vi "GUI_BELLA_ESP-2BL.vi"() -> ()   [LabVIEW 2020]
uses:
  Shared/GUI_Template/GUI_master/tcp_new_data_event.ctl
  Shared/GUI_Template/GUI_master/tcp new data cluster.ctl
panel:
  in  "Position.Axis 4::4":dbl=0.5 caption="M4A Vertical F4" min=-10000.0 max=10000.0 format="%_4f"
  in  "Position.Axis 3::4":dbl=0.5 caption="M4A Horizontal F3" min=-100000.0 max=100000.0 format="%_4f"
  in  "Position.Axis 2::4":dbl=0.5 caption="M2A Vertical F2" min=-10000.0 max=10000.0 format="%_4f"
  in  "Position.Axis 1::4":dbl=0.5 caption="M2A Horizontal F1" min=-100000.0 max=100000.0 format="%_4f"
  in  "Step size 1":dbl=100.0 caption="Step size" min=-22.0 max=22.0
  in  "GUIdevice 4":string="MCD-2BL-M4APicos"
  in  "Status.Axis 3::2":T1(ring) caption="Status"
  in  "Home.Axis 3::2":dbl=0.5 caption="Home" min=0.0 max=6.0 format="%_4f"
  in  "Power.Axis 3::2":enum16{"on", "off"}(ring) caption="Power"
  in  "Position.Axis 3::2":dbl=0.5 caption="Position" min=0.0 max=20.0 format="%_4f"
  in  "Status.Axis 3::3":T1(ring) caption="Status"
  in  "Home.Axis 3::3":dbl=0.5 caption="Home" min=0.0 max=6.0 format="%_4f"
  in  "Power.Axis 3::3":enum16{"on", "off"}(ring) caption="Power"
  in  "Position.Axis 3::3":dbl=0.5 caption="Position" min=0.0 max=20.0 format="%_4f"
  in  "Status.Axis 1::2":T1(ring) caption="Status"
  in  "Home.Axis 1::2":dbl=0.5 caption="Home" min=0.0 max=6.0 format="%_4f"
  in  "Power.Axis 1::2":enum16{"on", "off"}(ring) caption="Power"
  in  "Position.Axis 1::2":dbl=0.5 caption="Position" min=0.0 max=20.0 format="%_4f"
  in  "Status.Axis 2::2":T1(ring) caption="Status"
  in  "Home.Axis 2::2":dbl=0.5 caption="Home" min=0.0 max=6.0 format="%_4f"
  in  "Power.Axis 2::2":enum16{"on", "off"}(ring) caption="Power"
  in  "Position.Axis 2::2":dbl=0.5 caption="Position" min=0.0 max=20.0 format="%_4f"
  in  "Status.Axis 2::3":T1(ring) caption="Status"
  in  "Home.Axis 2::3":dbl=0.5 caption="Home" min=0.0 max=6.0 format="%_4f"
  in  "Power.Axis 2::3":enum16{"on", "off"}(ring) caption="Power"
  in  "Position.Axis 2::3":dbl=0.5 caption="Position" min=0.0 max=20.0 format="%_4f"
  in  "Status.Axis 1::3":T1(ring) caption="Status"
  in  "Home.Axis 1::3":dbl=0.5 caption="Home" min=0.0 max=6.0 format="%_4f"
  in  "Power.Axis 1::3":enum16{"on", "off"}(ring) caption="Power"
  in  "Position.Axis 1::3":dbl=0.5 caption="Position" min=0.0 max=20.0 format="%_4f"
  in  "Status.Axis 1::1":T1(ring) caption="Status"
  in  "Home.Axis 1::1":dbl=0.5 caption="Home" min=0.0 max=6.0 format="%_4f"
  in  "Power.Axis 1::1":enum16{"on", "off"}(ring) caption="Power"
  in  "Position.Axis 1::1":dbl=0.5 caption="Position" min=0.0 max=20.0 format="%_4f"
  in  "Status.Axis 2::1":T1(ring) caption="Status"
  in  "Home.Axis 2::1":dbl=0.5 caption="Home" min=0.0 max=6.0 format="%_4f"
  in  "Power.Axis 2::1":enum16{"on", "off"}(ring) caption="Power"
  in  "Position.Axis 2::1":dbl=0.5 caption="Position" min=0.0 max=20.0 format="%_4f"
  in  "stop":bool
  out "error IO 2":errorcluster
  out "tcp data event":T2
  in  "GUIdevice 3":string="MCD-2BL-ESPBTL3"
  in  "GUIdevice 1":string="MCD-2BL-ESPBTL1"
  in  "GUIdevice 2":string="MCD-2BL-ESPBTL2"
  in  "insert tag":bool=TRUE
  # "BELLA PW 2BL BTL MCD"
  # "F3M2 AXIS 1"
  # "Horizontal"
  # "Vertical"
  # "2BL PICOS"
  # "Horizontal"
  # "Vertical"
  # "F3M6 AXIS 1"
  # "F3M6 AXIS 2"
  # "Horizontal"
  # "Vertical"
  # "F3M5 AXIS 1"
  # "F3M5 AXIS 2"
  # "Horizontal"
  # "Vertical"
  # "F3M3 AXIS 2"
  # "F3M3 AXIS 1"
  # "F3M2 AXIS 2"
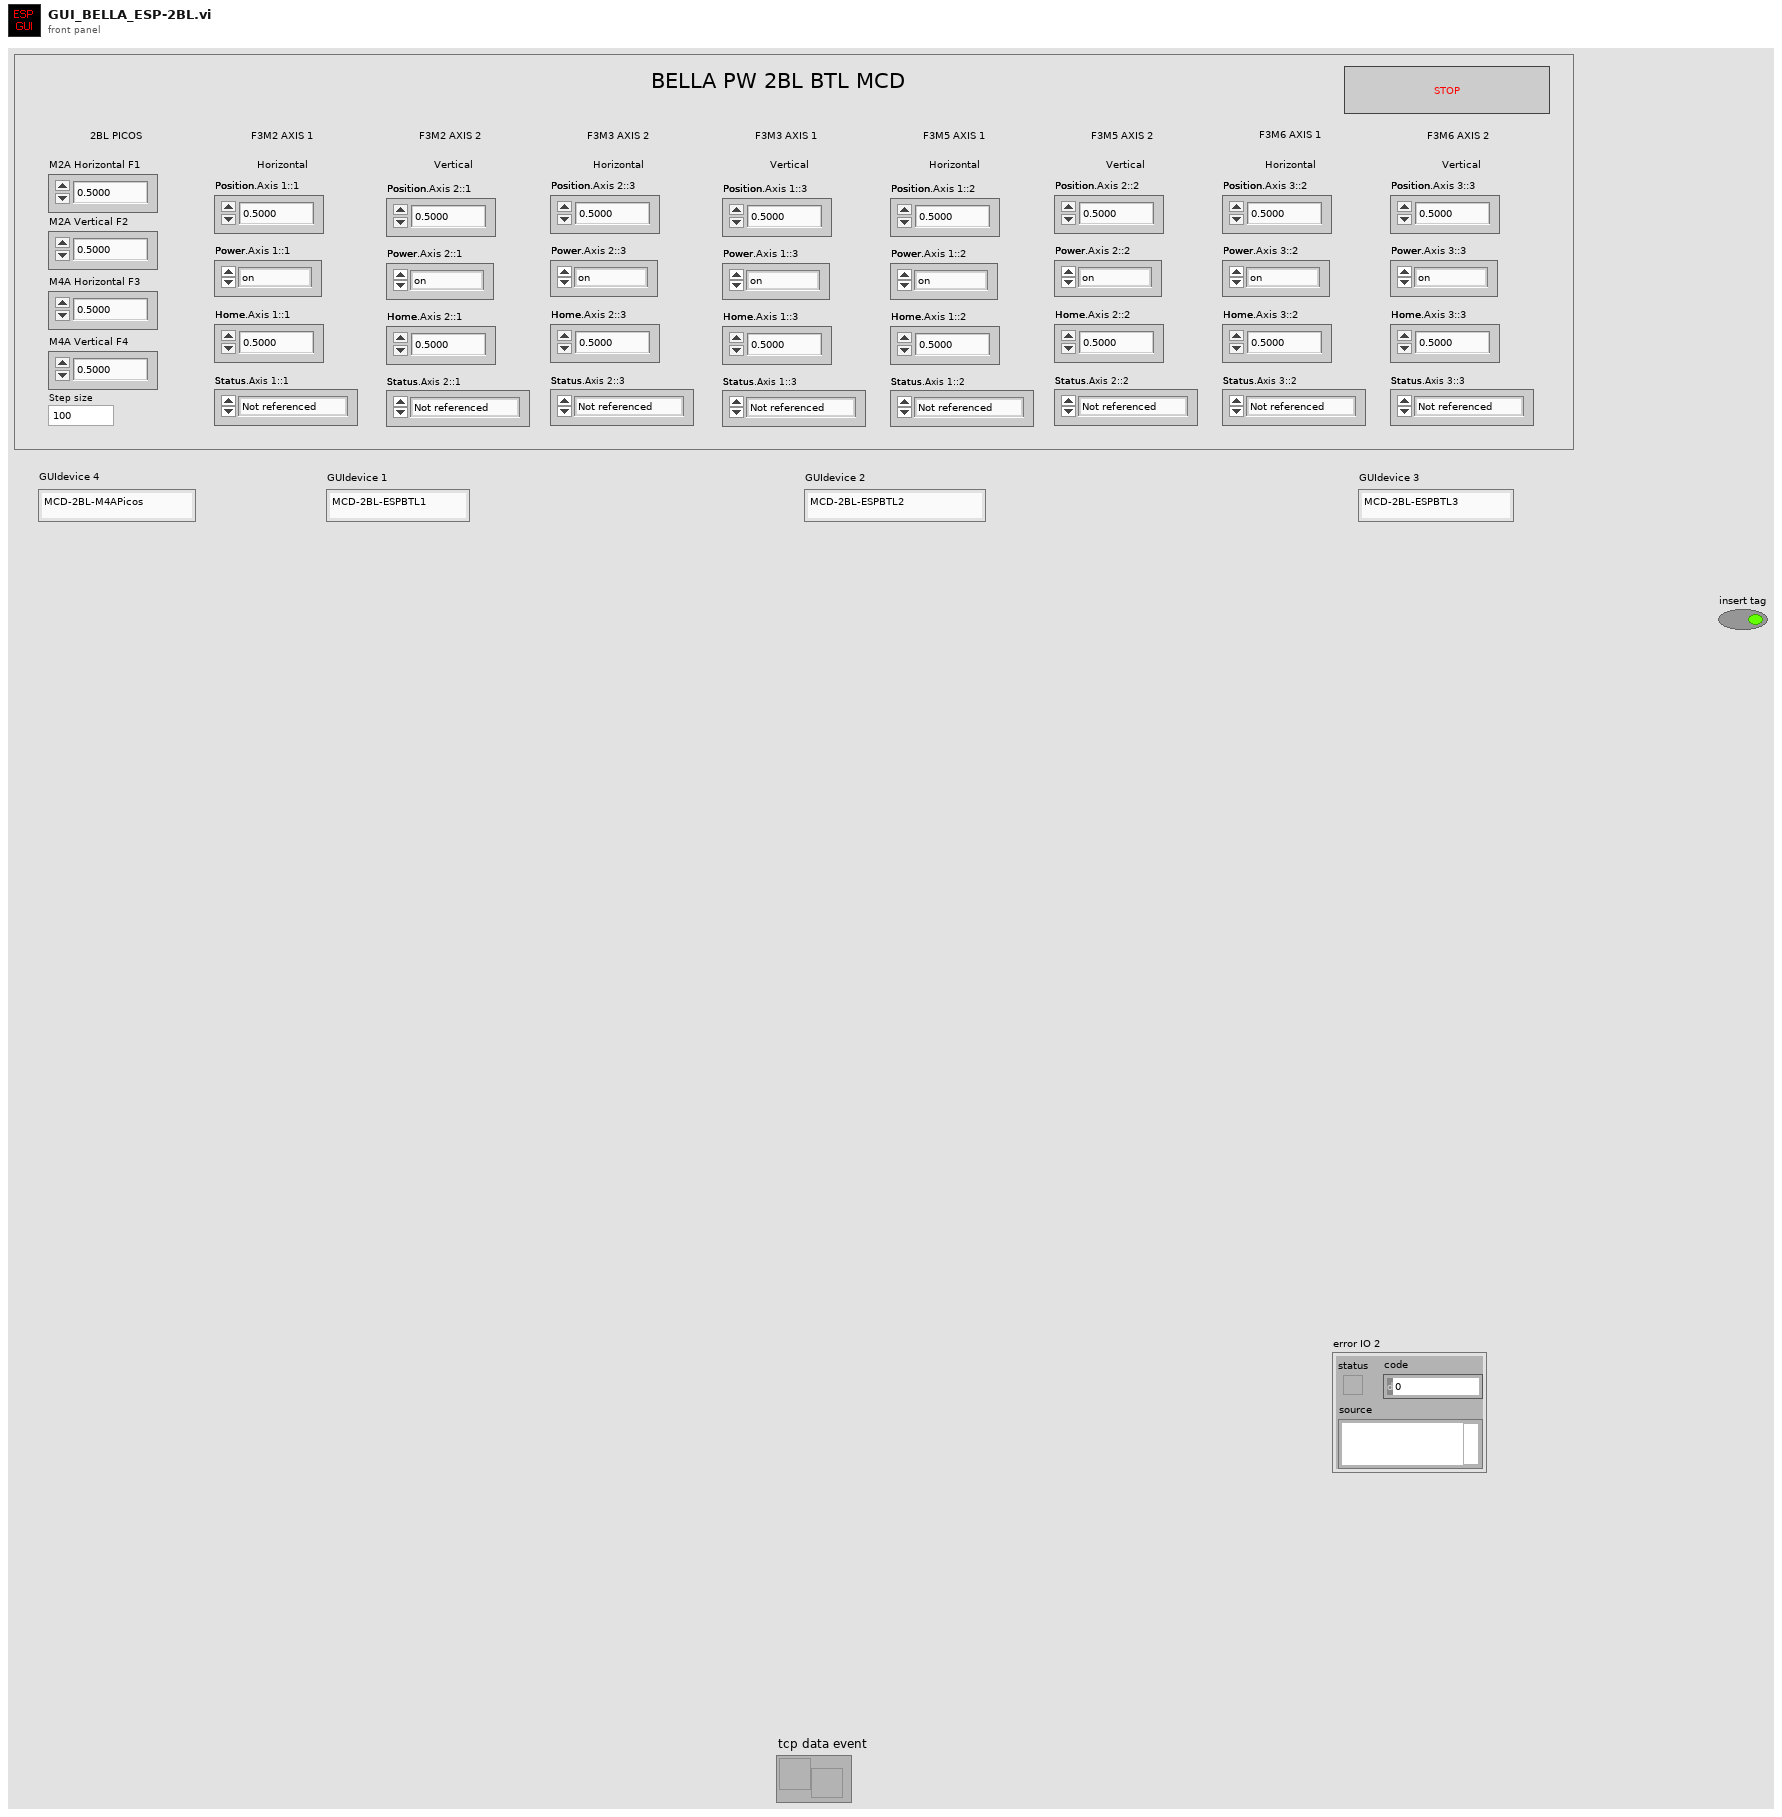
[diagram p1: front panel]
types:
  T1 = enum16{"Not referenced", "Homing", "Moving", "Ready"}
  T2 = typedef "tcp_new_data_event.ctl" = refnum<user-event>
  T3 = typedef "tcp new data cluster.ctl" = cluster{"EventEnum":enum16{"new data", "connection status update"}, "Device name":string}
  T4 = enum32{"Invalid", "Standard", "Closed", "Hidden", "Minimized", "Maximized"}
  T5 = enum32{"invalid app kind", "Development System", "Run Time System", "Student Edition", "Embedded LabVIEW", "Evaluation", "Custom"}
  T6 = cluster{"Core":cluster{"Current VI Reference":refnum<vi>, "Close Panel on Exit?":bool}, "Your Boolean data":bool, "Your string data":string}
  T7 = cluster{"Current VI Reference":refnum<vi>, "Close Panel on Exit?":bool}
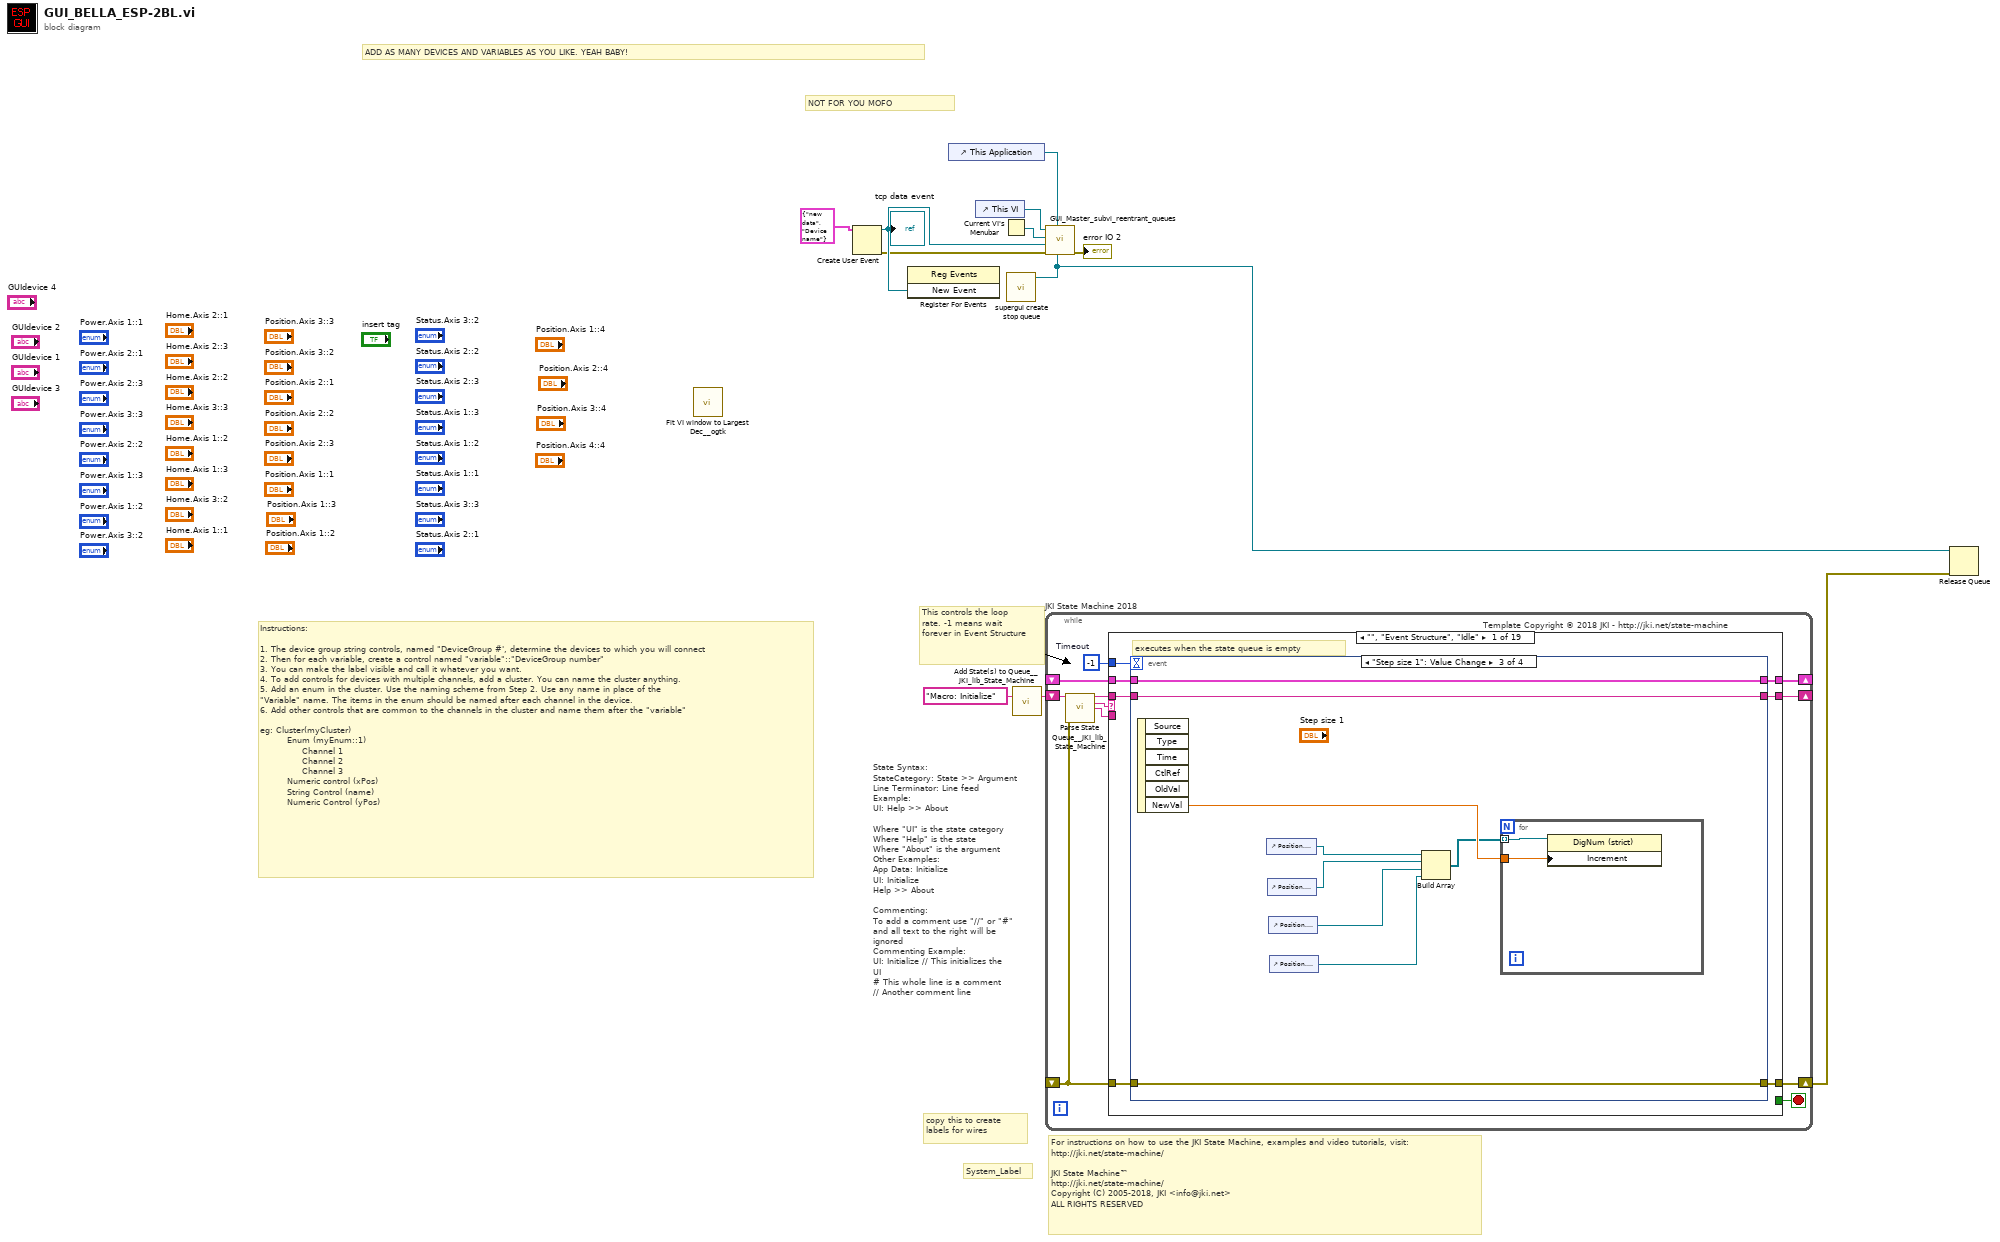
[diagram p0: block diagram]
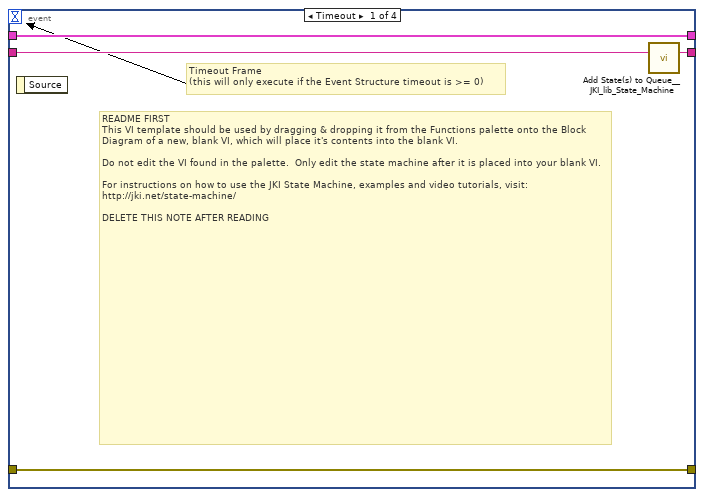
[diagram p2: hidden frame]
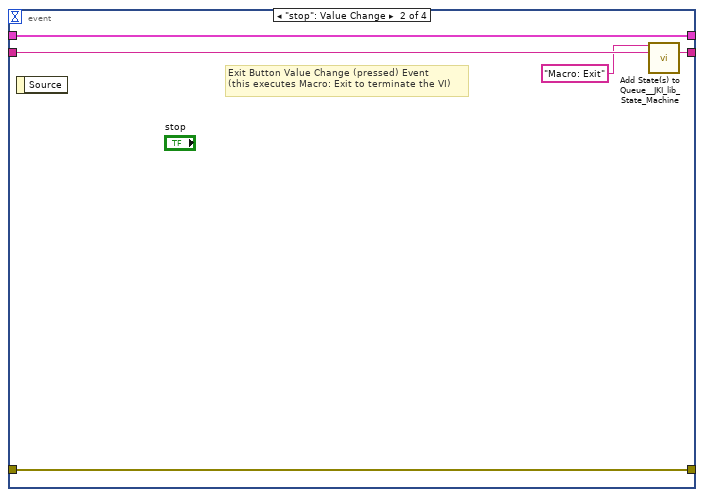
[diagram p3: hidden frame]
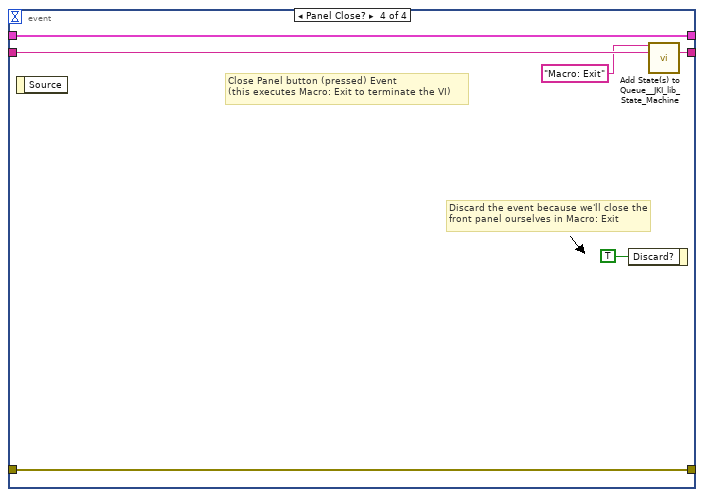
[diagram p4: hidden frame]
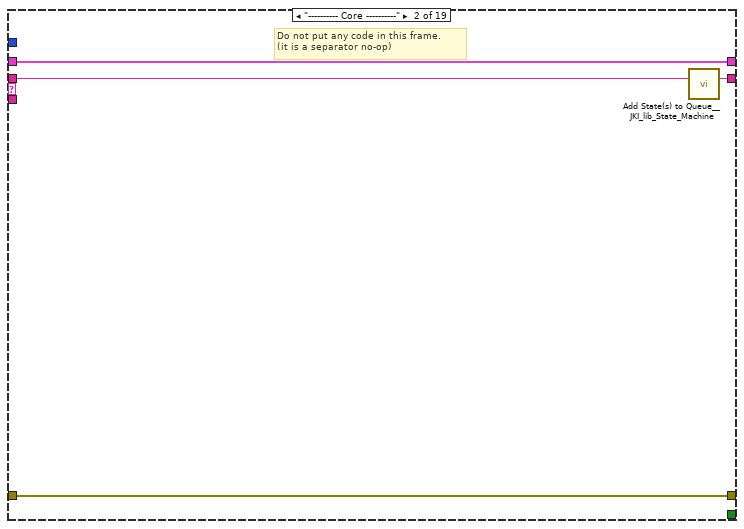
[diagram p5: hidden frame]
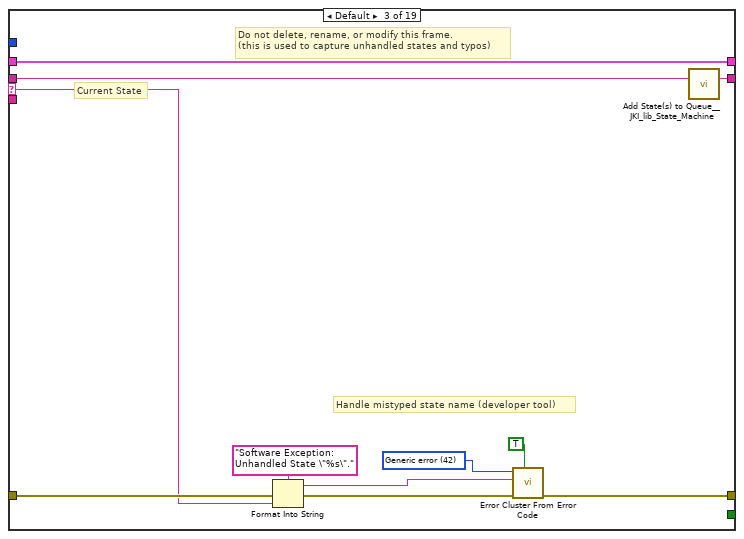
[diagram p6: hidden frame]
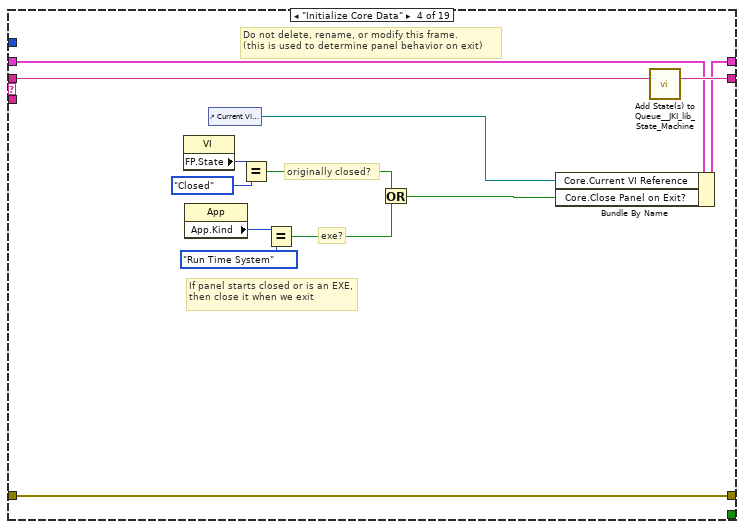
[diagram p7: hidden frame]
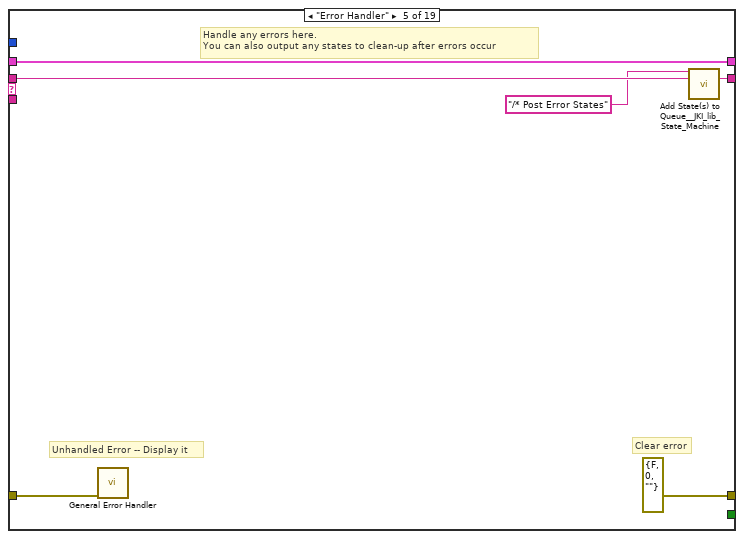
[diagram p8: hidden frame]
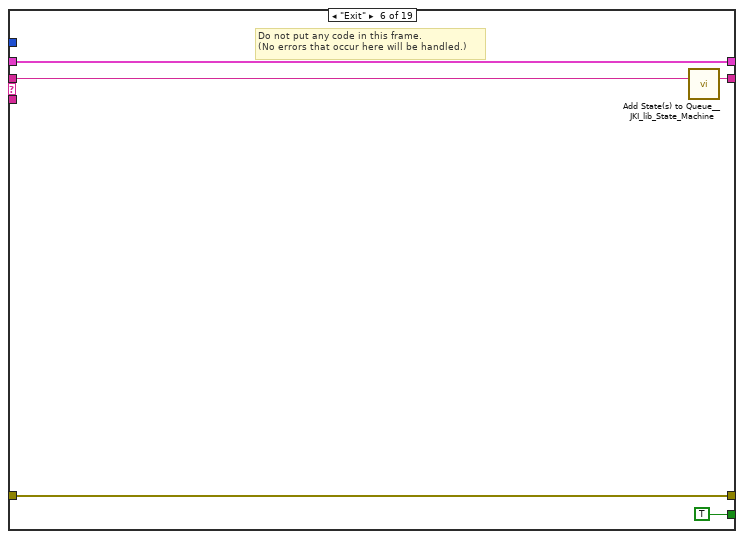
[diagram p9: hidden frame]
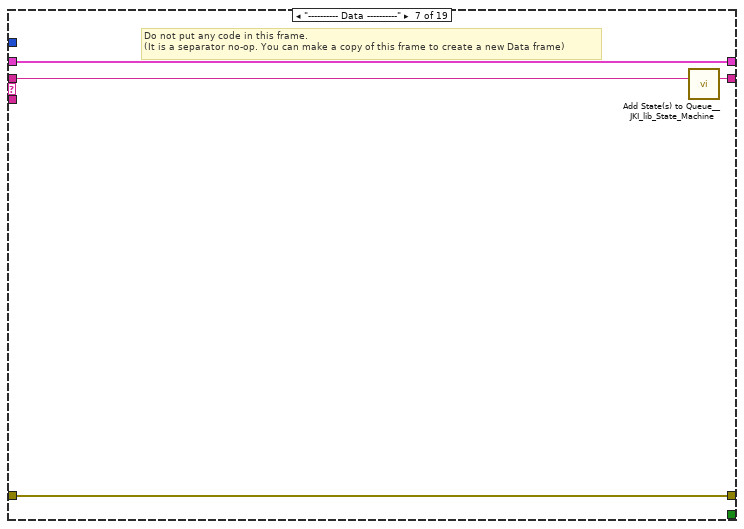
[diagram p10: hidden frame]
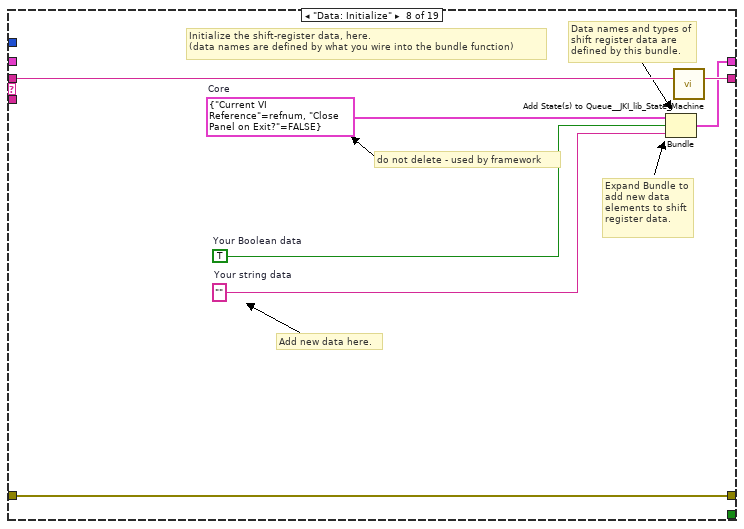
[diagram p11: hidden frame]
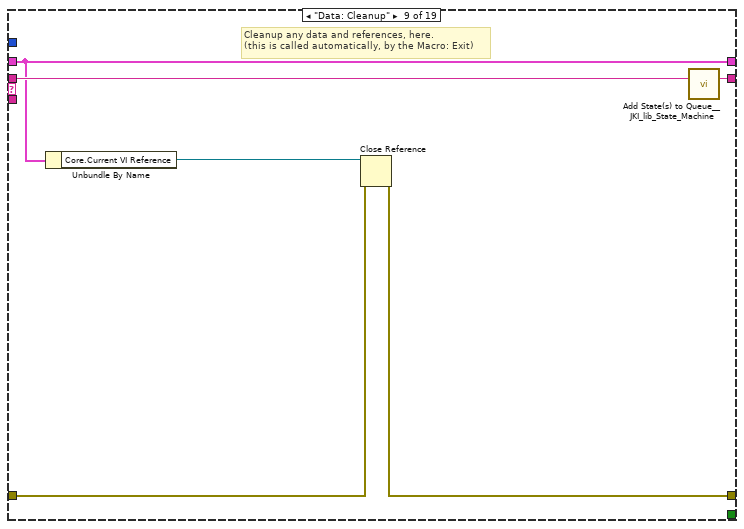
[diagram p12: hidden frame]
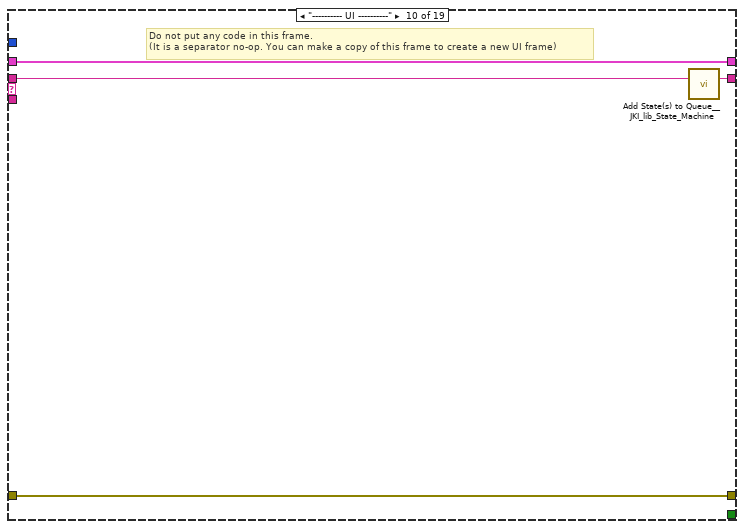
[diagram p13: hidden frame]
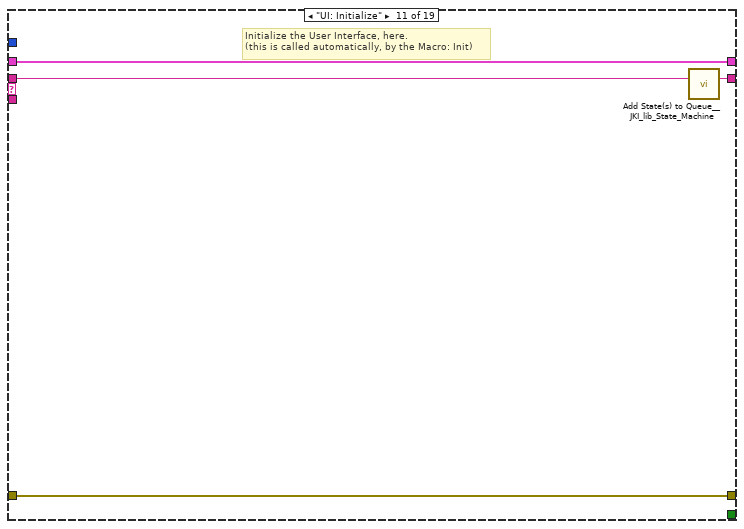
[diagram p14: hidden frame]
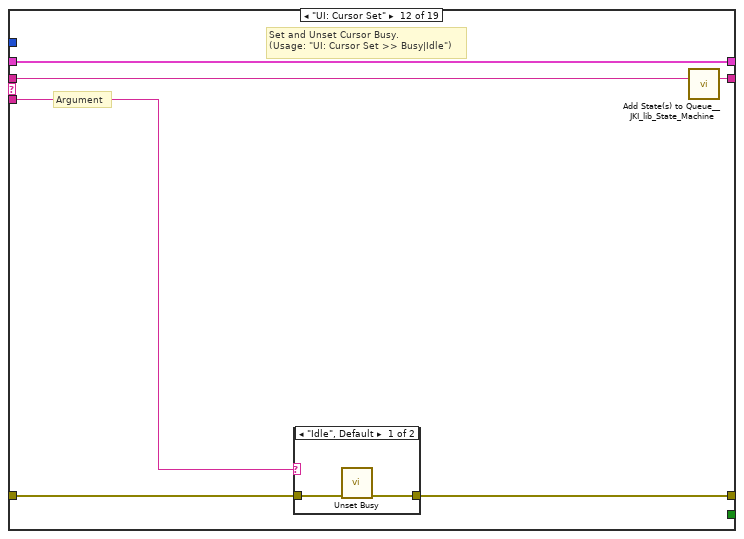
[diagram p15: hidden frame]
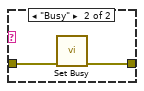
[diagram p16: hidden frame]
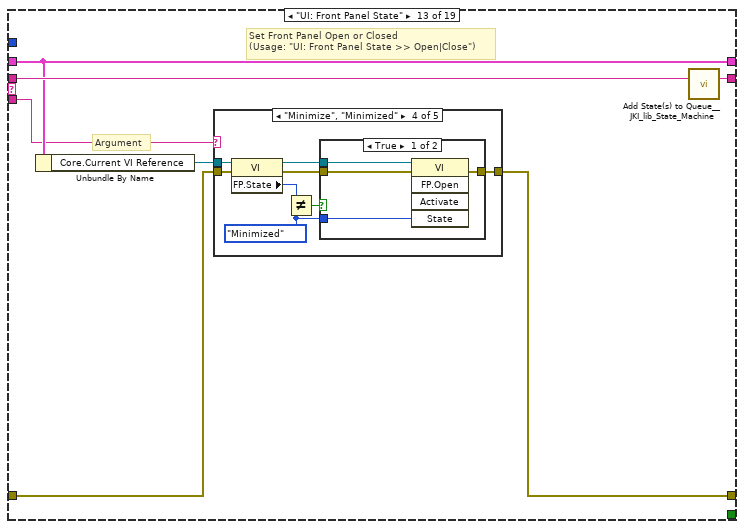
[diagram p17: hidden frame]
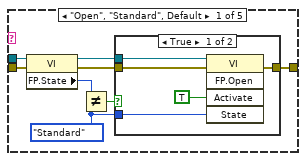
[diagram p18: hidden frame]
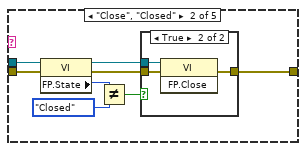
[diagram p20: hidden frame]
diagram:
  # "For instructions on how to use the JKI State Machine, examples and video tutorials, visit:\nhttp://jki.net/state-machine/\n\nJKI State Machine™\nhttp://jki.net/state-machine/\nCopyright (C) 2005-2018, JKI <info@jki.net>\nALL RIGHTS RESERVED"
  # "State Syntax:\nStateCategory: State >> Argument\nLine Terminator: Line feed\nExample:\nUI: Help >> About\n\nWhere \"UI\" is the state category\nWhere \"Help\" is the state\nWhere \"About\" is the argument\nOther Examples:\nApp Data: Initialize\nUI: Initialize\nHelp >> About\n\nCommenting:\nTo add a comment use \"//\" or \"#\" and all text to the right will be ignored\nCommenting Example:\nUI: Initialize // This initializes the UI\n# This whole line is a comment\n// Another comment line"
  # "copy this to create labels for wires"
  # "This controls the loop rate. -1 means wait forever in Event Structure"
  # "System_Label"
  # "NOT FOR YOU MOFO"
  # "Instructions:\n\n1. The device group string controls, named \"DeviceGroup #', determine the devices to which you will connect\n2. Then for each variable, create a control named \"variable\"::\"DeviceGroup number\"\n3. You can make the label visible and call it whatever you want.\n4. To add controls for devices with multiple channels, add a cluster. You can name the cluster anything.\n5. Add an enum in the cluster. Use the naming scheme from Step 2. Use any name in place of the \n\"Variable\" name. The items in the enum should be named after each channel in the device. \n6. Add other controls that are common to the channels in the cluster and name them after the \"variable\"\n\neg: Cluster(myCluster)\n         Enum (myEnum::1)\n              Channel 1 \n              Channel 2\n              Channel 3\n         Numeric control (xPos)\n         String Control (name)\n         Numeric Control (yPos)"
  # "ADD AS MANY DEVICES AND VARIABLES AS YOU LIKE. YEAH BABY!"
  n1 = call <userlib>:"Fit VI window to Largest Dec__ogtk.vi"() -> ()  [unwired: 6 in, 2 out]
  n2 = Create User Event(user event datatype=T3 {"EventEnum"=enum."new data", "Device name"="Device name"} ("New Event")) -> (user event=w10:refnum<user-event>, error out=w9:errorcluster)  [unwired: 1 in]
  "tcp data event" <- w10
  n3 = register-events(w10) -> ()  [unwired: 2 in, 2 out]
  n4 = control-ref of="This Application"() -> (w11:refnum<vi>)
  n5 = control-ref of="This VI"() -> (w6:refnum<vi>)
  n6 = Current VI's Menubar() -> (w7:refnum<k9>)
  n7 = call "supergui create stop queue.vi"() -> ("STOP Queue out"=w4:refnum<queue>)  [unwired: 11 in]
  n8 = call <vilib>:"Add State(s) to Queue__JKI_lib_State_Machine.vi"("State(s) in (\"\")"="Macro: Initialize") -> ("States Out"=w3:string)  [unwired: 14 in]
  n9 = call "GUI_Master_subvi_reentrant_queues.vi"("STOP Queue in"=w4, "This Application"=w11, "error in (no error)"=w9, "tcp data event"=w10, "Caller menu reference"=w7, "Caller VI ref"=w6) -> ("error out"=→"error IO 2":errorcluster)  [unwired: 5 in]
  n10 = while "JKI State Machine 2018" {
    shift-right: [w15] -> _
    shift-left: _ -> [w14]
    shift-right: [w18] -> w1
    shift-left: _ -> [w12]
    shift-right: [w17] -> _
    shift-left: w3 -> [w19]
    stop <- w16 stop-if-true
    w13 = -1  # Timeout
    # "Template Copyright © 2018 JKI - http://jki.net/state-machine"
    n11 = call <vilib>:"Parse State Queue__JKI_lib_State_Machine.vi"("State Queue"=w19, "Error In (no error)"=w12) -> ("Remaining States"=w21:string, "Current State"=w22:string, "Arguments"=w20:string)  [unwired: 11 in]
    n12 = case shown="\"\", \"Event Structure\", \"Idle\"" w22 {
      selector: w22 -> [_ _ w60 _ _ _ _ _ _ _ _ _ _ _ _ _ _ _ _]
      tunnel: w21 -> [w29 w59 w64 w83 w89 w94 w98 w105 w111 w115 w119 w125 w136 w205 w210 w220 w224 w228 w232]
      tunnel: w20 -> [_ _ _ _ _ _ _ _ _ _ _ w120 w130 _ _ _ _ _ _]
      tunnel: w14 -> [w27 w56 w62 w76 w86 w92 w95 _ w106 w112 w117 w123 w132 w202 w207 w217 w221 w225 w229]
      tunnel: [w26 w57 w66 w80 errorcluster {"status"=FALSE, "code"=0, "source"=""} ("error out") w91 w96 w102 w107 w113 w116 w121 w133 w203 w208 w218 w222 w226 w230] -> w18
      tunnel: w12 -> [w25 w57 w65 w80 w85 w91 w96 w102 w108 w113 w116 w122 w134 w203 w208 w218 w222 w226 w230]
      tunnel: [w28 w58 w63 w82 w88 w93 w97 w104 w110 w114 w118 w124 w135 w204 w209 w219 w223 w227 w231] -> w17
      tunnel: [_ _ _ _ _ TRUE _ _ _ _ _ _ _ _ _ _ _ _ _] -> w16
      tunnel: [w24 w56 w62 w81 w86 w92 w95 w103 w106 w112 w117 w123 w132 w202 w207 w217 w221 w225 w229] -> w15
      tunnel: w13 -> [w23 _ _ _ _ _ _ _ _ _ _ _ _ _ _ _ _ _ _]
      frame "", "Event Structure", "Idle" {
        # "executes when the state queue is empty"
        n13 = event shown="[2] \"Step size 1\": Value Change" {
          selector: _ -> [_ _ _ _]
          dyn-events: _ -> [_ _ _ _]
          timeout: w23 -> [_ _ _ _]
          tunnel: w29 -> [w33 w38 w40 w55]
          tunnel: [w32 w37 w40 w54] -> w28
          tunnel: w27 -> [w30 w35 w41 w52]
          tunnel: [w31 w36 w39 w53] -> w26
          tunnel: w25 -> [w31 w36 w39 w53]
          tunnel: [w30 w35 w41 w52] -> w24
          event Timeout {
            # "README FIRST\nThis VI template should be used by dragging & dropping it from the Functions palette onto the Block Diagram of a new, blank VI, which will place it's contents into the blank VI.\n\nDo not edit the VI found in the palette.  Only edit the state machine after it is placed into your blank VI.\n\nFor instructions on how to use the JKI State Machine, examples and video tutorials, visit:\nhttp://jki.net/state-machine/\n\nDELETE THIS NOTE AFTER READING"
            # "Timeout Frame\n(this will only execute if the Event Structure timeout is >= 0)"
            n14 = event-data() -> ()  [unwired: 1 in, 1 out]
            n15 = call <vilib>:"Add State(s) to Queue__JKI_lib_State_Machine.vi"("State(s) in (\"\")"=w33) -> ("States Out"=w32:string)  [unwired: 14 in]
          }
          event "stop": Value Change {
            # "Exit Button Value Change (pressed) Event\n(this executes Macro: Exit to terminate the VI)"
            n16 = event-data() -> ()  [unwired: 1 in, 1 out]
            n17 = call <vilib>:"Add State(s) to Queue__JKI_lib_State_Machine.vi"("State(s) in Front (\"\")"="Macro: Exit", "State(s) in (\"\")"=w38) -> ("States Out"=w37:string)  [unwired: 13 in]
          }
          event "Step size 1": Value Change {
            n18 = event-data() -> ("NewVal"=w43:dbl)  [unwired: 1 in, 5 out]
            n19 = control-ref of="Position.Axis 1::4"() -> (w47:refnum<vi>)
            n20 = control-ref of="Position.Axis 2::4"() -> (w46:refnum<vi>)
            n21 = control-ref of="Position.Axis 3::4"() -> (w45:refnum<vi>)
            n22 = control-ref of="Position.Axis 4::4"() -> (w44:refnum<vi>)
            n23 = Build Array(w47, w46, w45, w44) -> (w42:refnum<vi>[])
            n24 = for {
              tunnel: w43 -> [w49]
              tunnel: w42 -> [w48] mode=indexing
              n25 = property on="Property Node" class="DigNum (strict)"(reference=w48, "Increment"=w49) -> ()  [unwired: 1 in, 2 out]
            }
          }
          event Panel Close? {
            # "Discard the event because we'll close the front panel ourselves in Macro: Exit"
            # "Close Panel button (pressed) Event\n(this executes Macro: Exit to terminate the VI)"
            n26 = event-data() -> ()  [unwired: 1 in, 1 out]
            n27 = event-data("Discard?"=TRUE) -> ()  [unwired: 1 in, 1 out]
            n28 = call <vilib>:"Add State(s) to Queue__JKI_lib_State_Machine.vi"("State(s) in Front (\"\")"="Macro: Exit", "State(s) in (\"\")"=w55) -> ("States Out"=w54:string)  [unwired: 13 in]
          }
        }
      }
      frame "---------- Core ----------" {
        # "Do not put any code in this frame.\n(it is a separator no-op)"
        n29 = call <vilib>:"Add State(s) to Queue__JKI_lib_State_Machine.vi"("State(s) in (\"\")"=w59) -> ("States Out"=w58:string)  [unwired: 14 in]
      }
      frame Default {
        w69 = 42 items=["No error", "Argument error", "Memory is full", "Out of zone", "End of file", "File already open", "Generic file I/O error", "File not found", "File permission error", "Disk is full", "Duplicate path", "Too many files open", "System feature not enabled", "Resource file not found", "Cannot add resource", "Resource not found", "Image not found", "Image memory error", "Pen does not exist", "Config type invalid", "Config token not found", "Config parse error", "Config memory error", "Bad external code format", "Bad external code offset", "External code not present", "Null window", "Destroy window error", "Null menu", "Print aborted", "Bad print record", "Print driver error", "Windows error during printing", "Memory error during printing", "Print dialog error", "Generic print error", "Invalid device refnum", "Device not found", "Device parameter error", "Device unit error", "Cannot open device", "Device call aborted", "Generic error", "Cancelled by user", "Object ID too low", "Object ID too high", "Object not in heap", "Unknown heap", "Unknown object (invalid DefProc)", "Unknown object (DefProc not in table)", "Message out of range", "Invalid (null) method", "Unknown message", "Manager call not supported", "Bad address", "Network operation in progress", "Network operation timed out", "Connection is busy", "Network attribute not supported", "Network error", "Address in use", "System out of memory", "Connection aborted", "Connection refused", "Not connected", "Already connected", "Connection closed", "Initialization error (interapplication manager)", "Bad occurrence", "Wait on unbound occurrence handler", "Occurrence queue overflow", "Datalog type conflict", "Unused", "Unrecognized type (interapplication manager)", "Memory corrupt", "Failed to make temporary DLL", "Old CIN version", "Drag socket not found", "Failed to load drop-object", "Failed to register OLE object", "Failed to release OLE object", "Format specifier type mismatch", "Unknown format specifier", "Too few format specifiers", "Too many format specifiers", "Scan failed", "Newer CIN version", "Error converting to variant", "Runtime menu error", "Password tampered", "Variant attribute not found", "Incompatible variant data type", "Event data is not available", "Event Store is not present", "Occurrence is not found", "Event Queue is not created", "Event info is not available", "Refnum passed is NULL", "Error retrieving Class GUID", "Error retrieving CoClass GUID", "Error retrieving TypeLib GUID.", "Bad built application magic bytes.", "Specific driver is different from the specific driver associated with the Logical Name.", "There is no session opened to the class driver.", "Max Error", "MAX - Error with config objects", "MAX - Error loading configuration", "MAX - Group not supported"]
        # "Current State"
        # "Do not delete, rename, or modify this frame.\n(this is used to capture unhandled states and typos)"
        # "Handle mistyped state name (developer tool)"
        n30 = Format Into String(format string="Software Exception: Unhandled State \"%s\"." ("message"), error in=w65, w60) -> (resulting string=w68:string, error out=w67:errorcluster)  [unwired: 1 in]
        n31 = call <vilib>:"Error Cluster From Error Code.vi"("show call chain? (False)"=TRUE, "error in (no error)"=w67, "error message (\"\")"=w68, "error code (0)"=w69) -> ("error out"=w66:errorcluster)  [unwired: 5 in]
        n32 = call <vilib>:"Add State(s) to Queue__JKI_lib_State_Machine.vi"("State(s) in (\"\")"=w64) -> ("States Out"=w63:string)  [unwired: 14 in]
      }
      frame "Initialize Core Data" {
        # "Do not delete, rename, or modify this frame.\n(this is used to determine panel behavior on exit)"
        # "originally closed?"
        # "exe?"
        # "If panel starts closed or is an EXE, then close it when we exit"
        n33 = property class="VI"() -> ("FP.State"=w73:T4)  [unwired: 2 in, 2 out]
        n34 = property class="App"() -> ("App.Kind"=w79:T5)  [unwired: 2 in, 2 out]
        n35 = control-ref of="Current VI Reference"() -> (w74:refnum<vi>)
        n36 = Equal?(x=w73, y=T4."Closed" ("Front Panel Window:State")) -> (x = y?=w71:bool)
        n37 = Equal?(x=w79, y=T5."Run Time System" ("Application:Kind")) -> (x = y?=w77:bool)
        n38 = Or(x=w71, y=w77) -> (x .or. y?=w75:bool)
        n39 = Bundle By Name(cluster=w76, "Core.Current VI Reference"=w74, "Core.Close Panel on Exit?"=w75) -> (w81:T6)
        n40 = call <vilib>:"Add State(s) to Queue__JKI_lib_State_Machine.vi"("State(s) in (\"\")"=w83) -> ("States Out"=w82:string)  [unwired: 14 in]
      }
      frame "Error Handler" {
        # "Unhandled Error -- Display it"
        # "Handle any errors here.\nYou can also output any states to clean-up after errors occur"
        # "Clear error"
        n41 = call <vilib>:"General Error Handler.vi"("error in (no error)"=w85) -> ()  [unwired: 10 in, 5 out]
        n42 = call <vilib>:"Add State(s) to Queue__JKI_lib_State_Machine.vi"("State(s) in Front (\"\")"="/* Post Error States", "State(s) in (\"\")"=w89) -> ("States Out"=w88:string)  [unwired: 13 in]
      }
      frame "Exit" {
        # "Do not put any code in this frame.\n(No errors that occur here will be handled.)"
        n43 = call <vilib>:"Add State(s) to Queue__JKI_lib_State_Machine.vi"("State(s) in (\"\")"=w94) -> ("States Out"=w93:string)  [unwired: 14 in]
      }
      frame "---------- Data ----------" {
        # "Do not put any code in this frame.\n(It is a separator no-op. You can make a copy of this frame to create a new Data frame)"
        n44 = call <vilib>:"Add State(s) to Queue__JKI_lib_State_Machine.vi"("State(s) in (\"\")"=w98) -> ("States Out"=w97:string)  [unwired: 14 in]
      }
      frame "Data: Initialize" {
        w99 = T7 {"Current VI Reference"=refnum, "Close Panel on Exit?"=FALSE}  # Core
        w101 = TRUE  # Your Boolean data
        w100 = ""  # Your string data
        # "do not delete - used by framework"
        # "Expand Bundle to add new data elements to shift register data."
        # "Add new data here."
        # "Data names and types of shift register data are defined by this bundle."
        # "Initialize the shift-register data, here.\n(data names are defined by what you wire into the bundle function)"
        n45 = Bundle("Core"=w99, "Your Boolean data"=w101, "Your string data"=w100) -> (w103:T6)  [unwired: 1 in]
        n46 = call <vilib>:"Add State(s) to Queue__JKI_lib_State_Machine.vi"("State(s) in (\"\")"=w105) -> ("States Out"=w104:string)  [unwired: 14 in]
      }
      frame "Data: Cleanup" {
        # "Cleanup any data and references, here.\n(this is called automatically, by the Macro: Exit)"
        n47 = Unbundle By Name(w106) -> ("Core.Current VI Reference"=w109:refnum<vi>)
        n48 = Close Reference(reference=w109, error in (no error)=w108) -> (error out=w107:errorcluster)
        n49 = call <vilib>:"Add State(s) to Queue__JKI_lib_State_Machine.vi"("State(s) in (\"\")"=w111) -> ("States Out"=w110:string)  [unwired: 14 in]
      }
      frame "---------- UI ----------" {
        # "Do not put any code in this frame.\n(It is a separator no-op. You can make a copy of this frame to create a new UI frame)"
        n50 = call <vilib>:"Add State(s) to Queue__JKI_lib_State_Machine.vi"("State(s) in (\"\")"=w115) -> ("States Out"=w114:string)  [unwired: 14 in]
      }
      frame "UI: Initialize" {
        # "Initialize the User Interface, here.\n(this is called automatically, by the Macro: Init)"
        n51 = call <vilib>:"Add State(s) to Queue__JKI_lib_State_Machine.vi"("State(s) in (\"\")"=w119) -> ("States Out"=w118:string)  [unwired: 14 in]
      }
      frame "UI: Cursor Set" {
        # "Argument"
        # "Set and Unset Cursor Busy.\n(Usage: \"UI: Cursor Set >> Busy|Idle\")"
        n52 = case shown="\"Idle\", Default" w120 {
          tunnel: w122 -> [w127 w129]
          tunnel: [w126 w128] -> w121
          frame "Idle", Default {
            n53 = call <vilib>:"Unset Busy.vi"("error in (no error)"=w127) -> ("error out"=w126:errorcluster)  [unwired: 10 in]
          }
          frame "Busy" {
            n54 = call <vilib>:"Set Busy.vi"("error in (no error)"=w129) -> ("error out"=w128:errorcluster)  [unwired: 9 in, 1 out]
          }
        }
        n55 = call <vilib>:"Add State(s) to Queue__JKI_lib_State_Machine.vi"("State(s) in (\"\")"=w125) -> ("States Out"=w124:string)  [unwired: 14 in]
      }
      frame "UI: Front Panel State" {
        # "Argument"
        # "Set Front Panel Open or Closed\n(Usage: \"UI: Front Panel State >> Open|Close\")"
        n56 = Unbundle By Name(w132) -> ("Core.Current VI Reference"=w131:refnum<vi>)
        n57 = case shown="\"Minimize\", \"Minimized\"" w130 {
          tunnel: w134 -> [w142 w157 w168 w181 w194]
          tunnel: [w144 w158 w170 w183 w196] -> w133
          tunnel: w131 -> [w143 w155 w169 w182 w195]
          frame "Open", "Standard", Default {
            w137 = T4."Standard" ("State")
            n58 = property class="VI"(reference=w143, error in=w142) -> (reference out=w140:refnum<vi>, error out=w141:errorcluster, "FP.State"=w139:T4)
            n59 = Not Equal?(x=w139, y=w137) -> (x != y?=w138:bool)
            n60 = case shown="True" w138 {
              tunnel: [w148 w150] -> w144
              tunnel: w141 -> [w147 w150]
              tunnel: w140 -> [w146 _]
              tunnel: w137 -> [w145 _]
              frame True {
                n61 = invoke class="VI" method="FP.Open"(reference=w146, error in=w147, "Activate"=TRUE, "State"=w145) -> (error out=w148:errorcluster)  [unwired: 1 in, 4 out]
              }
              frame False {
              }
            }
          }
          frame "Close", "Closed" {
            n62 = property class="VI"(reference=w155, error in=w157) -> (reference out=w154:refnum<vi>, error out=w156:errorcluster, "FP.State"=w152:T4)
            n63 = Not Equal?(x=w152, y=T4."Closed" ("Front Panel Window:State")) -> (x != y?=w151:bool)
            n64 = case shown="True" w151 {
              tunnel: [w159 w162] -> w158
              tunnel: w156 -> [w159 w161]
              tunnel: w154 -> [_ w160]
              frame False {
              }
              frame True {
                n65 = invoke class="VI" method="FP.Close"(reference=w160, error in=w161) -> (error out=w162:errorcluster)  [unwired: 1 in, 2 out]
              }
            }
          }
          frame "Hidden", "Hide" {
            w163 = T4."Hidden" ("State")
            n66 = property class="VI"(reference=w169, error in=w168) -> (reference out=w166:refnum<vi>, error out=w167:errorcluster, "FP.State"=w165:T4)
            n67 = Not Equal?(x=w165, y=w163) -> (x != y?=w164:bool)
            n68 = case shown="True" w164 {
              tunnel: [w174 w175] -> w170
              tunnel: w167 -> [w173 w175]
              tunnel: w166 -> [w172 _]
              tunnel: w163 -> [w171 _]
              frame True {
                n69 = invoke class="VI" method="FP.Open"(reference=w172, error in=w173, "State"=w171) -> (error out=w174:errorcluster)  [unwired: 2 in, 4 out]
              }
              frame False {
              }
            }
          }
          frame "Minimize", "Minimized" {
            w176 = T4."Minimized" ("State")
            n70 = property class="VI"(reference=w182, error in=w181) -> (reference out=w179:refnum<vi>, error out=w180:errorcluster, "FP.State"=w178:T4)
            n71 = Not Equal?(x=w178, y=w176) -> (x != y?=w177:bool)
            n72 = case shown="True" w177 {
              tunnel: [w187 w188] -> w183
              tunnel: w180 -> [w186 w188]
              tunnel: w179 -> [w185 _]
              tunnel: w176 -> [w184 _]
              frame True {
                n73 = invoke class="VI" method="FP.Open"(reference=w185, error in=w186, "State"=w184) -> (error out=w187:errorcluster)  [unwired: 2 in, 4 out]
              }
              frame False {
              }
            }
          }
          frame "Maximize", "Maximized" {
            w189 = T4."Maximized" ("State")
            n74 = property class="VI"(reference=w195, error in=w194) -> (reference out=w192:refnum<vi>, error out=w193:errorcluster, "FP.State"=w191:T4)
            n75 = Not Equal?(x=w191, y=w189) -> (x != y?=w190:bool)
            n76 = case shown="True" w190 {
              tunnel: [w200 w201] -> w196
              tunnel: w193 -> [w199 w201]
              tunnel: w192 -> [w198 _]
              tunnel: w189 -> [w197 _]
              frame True {
                n77 = invoke class="VI" method="FP.Open"(reference=w198, error in=w199, "State"=w197) -> (error out=w200:errorcluster)  [unwired: 2 in, 4 out]
              }
              frame False {
              }
            }
          }
        }
        n78 = call <vilib>:"Add State(s) to Queue__JKI_lib_State_Machine.vi"("State(s) in (\"\")"=w136) -> ("States Out"=w135:string)  [unwired: 14 in]
      }
      frame "---------- Macro ----------" {
        # "Do not put any code in this frame.\n(It is a separator no-op. You can make a copy of this frame to create a new Macro frame)"
        n79 = call <vilib>:"Add State(s) to Queue__JKI_lib_State_Machine.vi"("State(s) in (\"\")"=w205) -> ("States Out"=w204:string)  [unwired: 14 in]
      }
      frame "Macro: Initialize" {
        w206 = "Data: Initialize\nInitialize Core Data\nUI: Initialize\nUI: Front Panel State >> Open"  # Data: Initialize Initialize Core Data UI: Initialize UI: Front Panel State >> Open
        # "Initialization Macro\n(This is called once, when the VI starts)"
        n80 = call <vilib>:"Add State(s) to Queue__JKI_lib_State_Machine.vi"("State(s) in Front (\"\")"=w206, "State(s) in (\"\")"=w210) -> ("States Out"=w209:string)  [unwired: 13 in]
      }
      frame "Macro: Exit" {
        # "Exit Macro\n(This is called once, when the VI exits)"
        n81 = Unbundle By Name(w217) -> ("Core.Close Panel on Exit?"=w216:bool)
        n82 = Select(t="UI: Front Panel State >> Close", s=w216, f="") -> (s? t:f=w213:string)
        n83 = call <vilib>:"Add State(s) to Queue__JKI_lib_State_Machine.vi"("State(s) in (\"\")"=w213, "State(s) at Back (\"\")"="Data: Cleanup\nExit") -> ("States Out"=w211:string)  [unwired: 13 in]
        n84 = call <vilib>:"Add State(s) to Queue__JKI_lib_State_Machine.vi"("State(s) in Front (\"\")"=w211, "State(s) in (\"\")"=w220) -> ("States Out"=w219:string)  [unwired: 13 in]
      }
      frame "---------- New Category ----------" {
        # "Template Separator\n(You can make a copy of, or modify, this frame)"
        n85 = call <vilib>:"Add State(s) to Queue__JKI_lib_State_Machine.vi"("State(s) in (\"\")"=w224) -> ("States Out"=w223:string)  [unwired: 14 in]
      }
      frame "New Category: 1" {
        # "Your code here.\n(You can make a copy of, or modify, this frame)"
        n86 = call <vilib>:"Add State(s) to Queue__JKI_lib_State_Machine.vi"("State(s) in (\"\")"=w228) -> ("States Out"=w227:string)  [unwired: 14 in]
      }
      frame "New Category: 2" {
        # "Your code here.\n(You can make a copy of, or modify, this frame)"
        n87 = call <vilib>:"Add State(s) to Queue__JKI_lib_State_Machine.vi"("State(s) in (\"\")"=w232) -> ("States Out"=w231:string)  [unwired: 14 in]
      }
    }
  }
  n88 = Release Queue(queue=w4, error in (no error)=w1) -> ()  [unwired: 1 in, 3 out]
